vi "MTS_CreateWriteMSW.vi"(7 "Rewrite":bool, 8 "error in (no error)":errorcluster, 9 "Comment":string, 10 "Files in Workspace":T1(array[cluster]), 11 "Workspace Path":path) -> (0 "error out":errorcluster, 1 "Created":string, 2 "Comment (dup)":string, 3 "Files in Workspace (dup)":T1(array[cluster]))   [LabVIEW 2013]
uses:
  <vilib>/Utility/config.llb/Read Key (String).vi
  <vilib>/Utility/config.llb/Write Key (String).vi
  <vilib>/Utility/config.llb/Write Key (Path).vi
  <vilib>/Utility/config.llb/Write Key (I32).vi
  <vilib>/Utility/config.llb/Write Key (Double).vi
  <vilib>/Utility/config.llb/Write Key (U32).vi
  <vilib>/Utility/config.llb/NI_LVConfig.lvlib
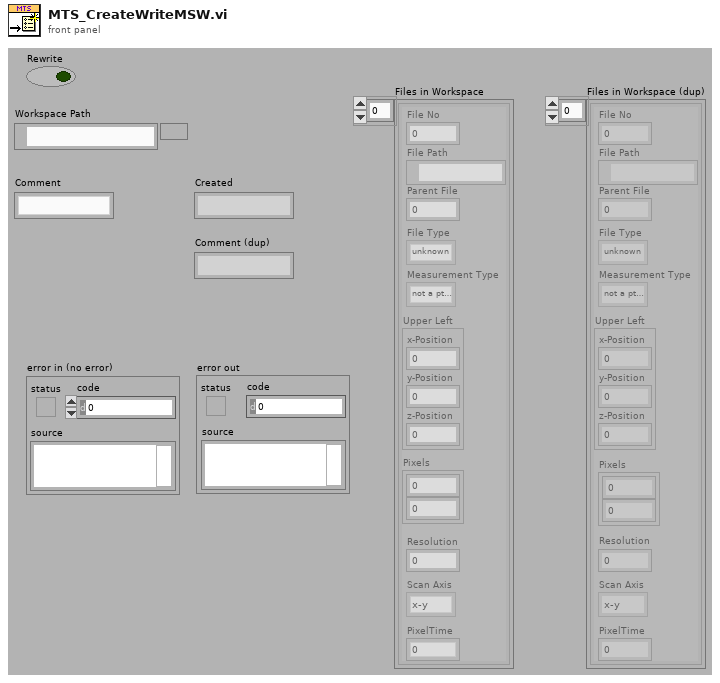
[diagram p1: front panel]
types:
  T1 = cluster{"File No":i32, "File Path":path, "Parent File":i32, "File Type":enum16{"unknown", "pt3 File", "png Image", "bmp Image"}, "Measurement Type":enum16{"not a pt3 File", "Image File", "Point Measurement", "Auto Point", "Line Scan", "Grid Scan"}, "Upper Left":cluster{"x-Position":dbl, "y-Position":dbl, "z-Position":dbl}, "Pixels":dbl[], "Resolution":dbl, "Scan Axis":enum32{"x-y", "x-z", "y-x", "y-z", "z-x", "z-y"}, "PixelTime":dbl}[]
  T2 = typedef "NI_LVConfig.lvlib/Config Data RefNum.ctl" = refnum<k1>
  T3 = enum16{"unknown", "pt3 File", "png Image", "bmp Image"}
  T4 = enum16{"not a pt3 File", "Image File", "Point Measurement", "Auto Point", "Line Scan", "Grid Scan"}
  T5 = cluster{"x-Position":dbl, "y-Position":dbl, "z-Position":dbl}
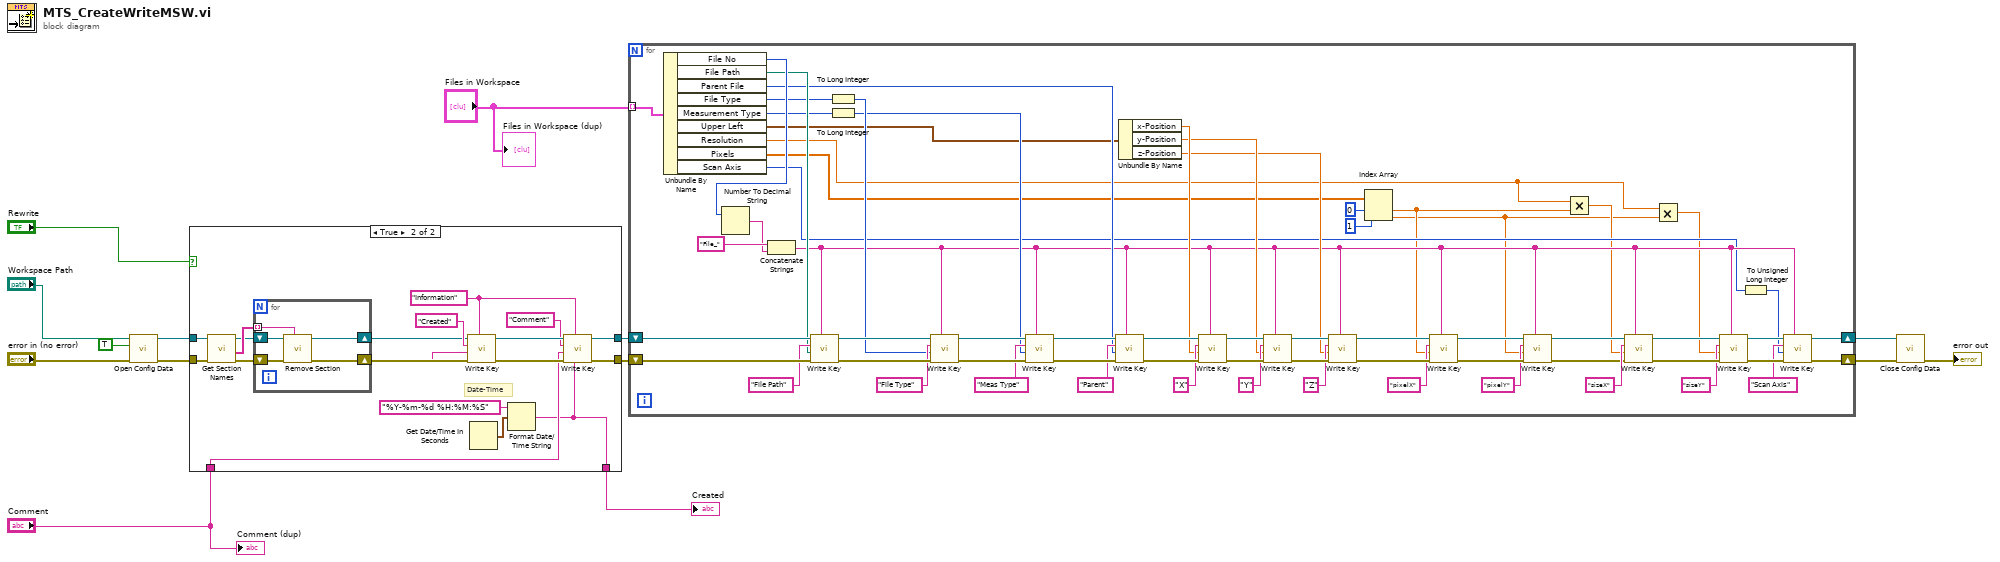
[diagram p0: block diagram]
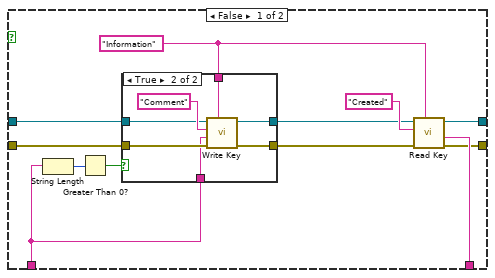
[diagram p2: hidden frame]
diagram:
  n1 = call <vilib>:"Open Config Data.vi"("error in (no error)"="error in (no error)", "create file if necessary (T)"=TRUE, "configuration file path"="Workspace Path") -> ("error out"=w11:errorcluster, "refnum"=w10:T2)  [unwired: 6 in, 1 out]
  n2 = case shown="True" "Rewrite" {
    tunnel: w11 -> [w22 w43]
    tunnel: w10 -> [w16 w42]
    tunnel: [w25 w41] -> w9
    tunnel: [w24 w40] -> w8
    tunnel: "Comment" -> [w17 w48]
    tunnel: [w26 w36] -> w2
    frame False {
      w20 = "Information" ("section")
      n3 = String Length(string=w17) -> (length=w19:i32)
      n4 = Greater Than 0?(x=w19) -> (x > 0?=w18:bool)
      n5 = case shown="True" w18 {
        tunnel: w22 -> [w27 w35]
        tunnel: [w27 w34] -> w21
        tunnel: w20 -> [_ w33]
        tunnel: w17 -> [_ w31]
        tunnel: w16 -> [w28 w30]
        tunnel: [w28 w29] -> w15
        frame False {
        }
        frame True {
          n6 = call-poly <vilib>:"Write Key.vi"("section"=w33, "error in (no error)"=w35, "value"=w31, "key"="Comment", "refnum"=w30) -> ("error out"=w34:errorcluster, "refnum out"=w29:T2)  [unwired: 4 in, 1 out]
        }
      }
      n7 = call-poly <vilib>:"Read Key.vi"("section"=w20, "error in (no error)"=w21, "key"="Created", "refnum"=w15) -> ("error out"=w25:errorcluster, "value"=w26:string, "refnum out"=w24:T2)  [unwired: 4 in, 1 out]
    }
    frame True {
      w50 = "Information" ("section")
      # "Date-Time"
      n8 = call <vilib>:"Get Section Names.vi"("error in (no error)"=w43, "refnum"=w42) -> ("error out"=w45:errorcluster, "section names"=w44:string[], "refnum out"=w39:T2)  [unwired: 7 in]
      n9 = for {
        tunnel: w44 -> [w56] mode=indexing
        shift-right: [w54] -> w37
        shift-left: w45 -> [w57]
        shift-right: [w55] -> w38
        shift-left: w39 -> [w58]
        n10 = call <vilib>:"Remove Section.vi"("section"=w56, "error in (no error)"=w57, "refnum"=w58) -> ("error out"=w54:errorcluster, "refnum out"=w55:T2)  [unwired: 6 in, 1 out]
      }
      n11 = Get Date/Time In Seconds() -> (seconds since 1Jan1904=w47:timestamp)
      n12 = Format Date/Time String(time format string (%c)="%Y-%m-%d %H:%M:%S", seconds (now)=w47) -> (date/time string=w36:string)  [unwired: 1 out]
      n13 = call-poly <vilib>:"Write Key.vi"("section"=w50, "error in (no error)"=w37, "value"=w36, "key"="Created", "refnum"=w38) -> ("error out"=w52:errorcluster, "refnum out"=w51:T2)  [unwired: 4 in, 1 out]
      n14 = call-poly <vilib>:"Write Key.vi"("section"=w50, "error in (no error)"=w52, "value"=w48, "key"="Comment", "refnum"=w51) -> ("error out"=w41:errorcluster, "refnum out"=w40:T2)  [unwired: 4 in, 1 out]
    }
  }
  "Created" <- w2
  n15 = for {
    shift-right: [w70] -> w7
    shift-left: w9 -> [w121]
    tunnel: "Files in Workspace" -> [w86] mode=indexing
    shift-right: [w69] -> w1
    shift-left: w8 -> [w120]
    n16 = Unbundle By Name(w86) -> ("File No"=w85:i32, "File Path"=w84:path, "Parent File"=w83:i32, "File Type"=w82:T3, "Measurement Type"=w80:T4, "Upper Left"=w78:T5, "Resolution"=w59:dbl, "Pixels"=w72:dbl[], "Scan Axis"=w65:enum32{"x-y", "x-z", "y-x", "y-z", "z-x", "z-y"})
    n17 = Number To Decimal String(number=w85) -> (decimal integer string=w87:string)  [unwired: 1 in]
    n18 = Concatenate Strings("File_" ("regular expression"), w87) -> (w67:string)
    n19 = call-poly <vilib>:"Write Key.vi"("section"=w67, "error in (no error)"=w121, "value"=w84, "key"="File Path", "refnum"=w120) -> ("error out"=w118:errorcluster, "refnum out"=w117:T2)  [unwired: 4 in, 1 out]
    n20 = To Long Integer(number=w82) -> (32bit integer=w81:i32)
    n21 = To Long Integer(number=w80) -> (32bit integer=w79:i32)
    n22 = call-poly <vilib>:"Write Key.vi"("section"=w67, "error in (no error)"=w118, "value"=w81, "key"="File Type", "refnum"=w117) -> ("error out"=w115:errorcluster, "refnum out"=w114:T2)  [unwired: 4 in, 1 out]
    n23 = call-poly <vilib>:"Write Key.vi"("section"=w67, "error in (no error)"=w115, "value"=w79, "key"="Meas Type", "refnum"=w114) -> ("error out"=w113:errorcluster, "refnum out"=w112:T2)  [unwired: 4 in, 1 out]
    n24 = call-poly <vilib>:"Write Key.vi"("section"=w67, "error in (no error)"=w113, "value"=w83, "key"="Parent", "refnum"=w112) -> ("error out"=w109:errorcluster, "refnum out"=w103:T2)  [unwired: 4 in, 1 out]
    n25 = Unbundle By Name(w78) -> ("x-Position"=w77:dbl, "y-Position"=w76:dbl, "z-Position"=w75:dbl)
    n26 = call-poly <vilib>:"Write Key.vi"("section"=w67, "error in (no error)"=w109, "value"=w77, "key"="X", "refnum"=w103) -> ("error out"=w108:errorcluster, "refnum out"=w102:T2)  [unwired: 4 in, 1 out]
    n27 = call-poly <vilib>:"Write Key.vi"("section"=w67, "error in (no error)"=w108, "value"=w76, "key"="Y", "refnum"=w102) -> ("error out"=w107:errorcluster, "refnum out"=w101:T2)  [unwired: 4 in, 1 out]
    n28 = call-poly <vilib>:"Write Key.vi"("section"=w67, "error in (no error)"=w107, "value"=w75, "key"="Z", "refnum"=w101) -> ("error out"=w100:errorcluster, "refnum out"=w98:T2)  [unwired: 4 in, 1 out]
    n29 = Index Array(array=w72, index #1=0 ("index"), index #2=1 ("index")) -> (element #1=w63:dbl, element #2=w61:dbl)
    n30 = call-poly <vilib>:"Write Key.vi"("section"=w67, "error in (no error)"=w100, "value"=w63, "key"="pixelX", "refnum"=w98) -> ("error out"=w99:errorcluster, "refnum out"=w97:T2)  [unwired: 4 in, 1 out]
    n31 = call-poly <vilib>:"Write Key.vi"("section"=w67, "error in (no error)"=w99, "value"=w61, "key"="pixelY", "refnum"=w97) -> ("error out"=w90:errorcluster, "refnum out"=w89:T2)  [unwired: 4 in, 1 out]
    n32 = Multiply(x=w59, y=w63) -> (x*y=w62:dbl)
    n33 = call-poly <vilib>:"Write Key.vi"("section"=w67, "error in (no error)"=w90, "value"=w62, "key"="sizeX", "refnum"=w89) -> ("error out"=w94:errorcluster, "refnum out"=w93:T2)  [unwired: 4 in, 1 out]
    n34 = Multiply(x=w59, y=w61) -> (x*y=w60:dbl)
    n35 = call-poly <vilib>:"Write Key.vi"("section"=w67, "error in (no error)"=w94, "value"=w60, "key"="sizeY", "refnum"=w93) -> ("error out"=w71:errorcluster, "refnum out"=w68:T2)  [unwired: 4 in, 1 out]
    n36 = To Unsigned Long Integer(number=w65) -> (unsigned 32bit integer=w64:u32)
    n37 = call-poly <vilib>:"Write Key.vi"("section"=w67, "error in (no error)"=w71, "value"=w64, "key"="Scan Axis", "refnum"=w68) -> ("error out"=w70:errorcluster, "refnum out"=w69:T2)  [unwired: 4 in, 1 out]
  }
  n38 = call <vilib>:"Close Config Data.vi"("error in (no error)"=w7, "refnum"=w1) -> ("error out"=→"error out":errorcluster)  [unwired: 8 in, 1 out]
  "Comment (dup)" <- "Comment"
  "Files in Workspace (dup)" <- "Files in Workspace"
